vi "Memory.Pointer.New.vi"(7 "allocation limit (2^31: 2GiB)":u64=2147483647 format="%08x bytes", 8 "error in (no error)":errorcluster, 10 "size":u64 format="%d bytes") -> (0 "error out":errorcluster, 2 "allocated size":u64 format="%d bytes", 3 "Pointer out":refnum<class "Memory.Pointer.Void.lvclass">)   [LabVIEW 2016, in "LabVIEW Memory Manager.lvlib" / "Memory.Pointer.Void.lvclass"]
uses:
  Memory.Pointer.Void.lvclass
  Memory.Pointer.Void.lvclass/Memory.Pointer.Void.ctl
  Memory.Pointer.Set Address.vi
  Memory.Pointer.Set Size.vi
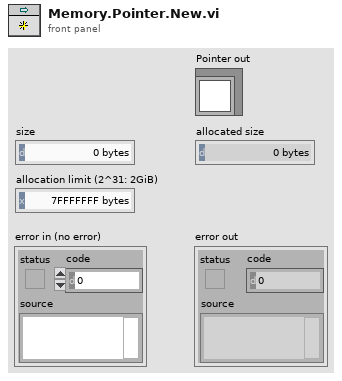
[diagram p1: front panel]
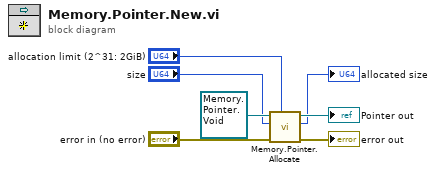
[diagram p0: block diagram]
diagram:
  n1 = call "Memory.Pointer.Allocate.vi"("allocation limit (2^31: 2GiB)"="allocation limit (2^31: 2GiB)", "error in (no error)"="error in (no error)", "size"="size", "Pointer in"=refnum<class "Memory.Pointer.Void.lvclass"> refnum) -> ("error out"=→"error out":errorcluster, "allocated size"=→"allocated size":u64, "Pointer out"=→"Pointer out":refnum<class "Memory.Pointer.Void.lvclass">)  [unwired: 5 in]
